vi "Data.Engine.Write Data to HW.vi"(8 "error in":errorcluster, 11 "Data Access API in":refnum<class "Data Access Engine (Express).lvclass">) -> (0 "error out":errorcluster, 3 "Data Access API out":refnum<class "Data Access Engine (Express).lvclass">)   [LabVIEW 2027, in "Data Access Engine (Express).lvlib" / "Data Access Engine (Express).lvclass"]
uses:
  Data Access Engine (Express).lvclass
  Data Access Engine (Express).lvclass/Data Access Engine (Express).ctl
  Access Type Classes/Read/Read.lvclass/Read.ctl
  <userlib>/Custom Device Interfaces_v1.lvlibp/CustomDeviceAPI/Custom Device API.lvclass
  Access Type Classes/Read/Read.lvclass
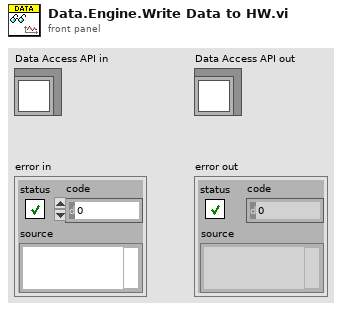
[diagram p1: front panel]
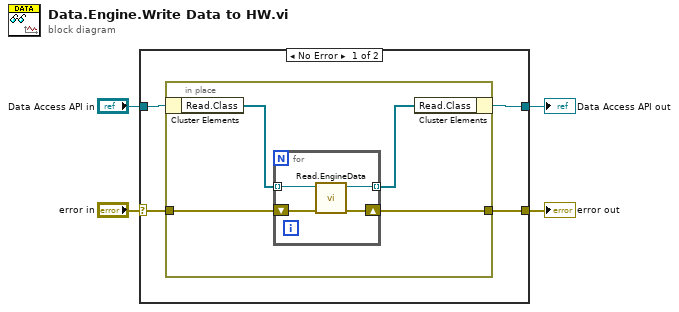
[diagram p0: block diagram]
diagram:
  n1 = case shown="No Error" "error in" {
    selector: "error in" -> [w6 w18]
    tunnel: [w8 w18] -> w3
    tunnel: [w7 w17] -> w1
    tunnel: "Data Access API in" -> [w5 w17]
    frame No Error {
      n2 = in-place {
        in-place-border: w6 -> [w9]
        in-place-border: [w12] -> w8
        n3 = in-place-cluster #1(w5) -> ("Read.Class"=w11:refnum<class "Read.lvclass">[])
        n4 = for {
          tunnel: w11 -> [w15] mode=indexing
          shift-right: [w14] -> w12
          shift-left: w9 -> [w16]
          tunnel: [w13] -> w10 mode=indexing
          n5 = call "Read.EngineData.vi"("error in"=w16, "Read in"=w15) -> ("error out"=w14:errorcluster, "Read out"=w13:refnum<class "Read.lvclass">)  [unwired: 8 in]
        }
        n6 = in-place-cluster #1("Read.Class"=w10) -> (w7:refnum<class "Data Access Engine (Express).lvclass">)
      }
    }
    frame Error {
    }
  }
  "error out" <- w3
  "Data Access API out" <- w1
